vi "Low Over Current Test 1.vi"(0 "Device Name":string="Dev4", 1 "Device/Ports/Lines":string="Dev1/port0/line1,Dev1/port0/line13,Dev1/port0/line6,Dev1/port0/line23,Dev1/port0/line17", 3 "error in":errorcluster) -> (10 "error out":errorcluster)   [LabVIEW 2015]
panel:
  # "True means close relay"
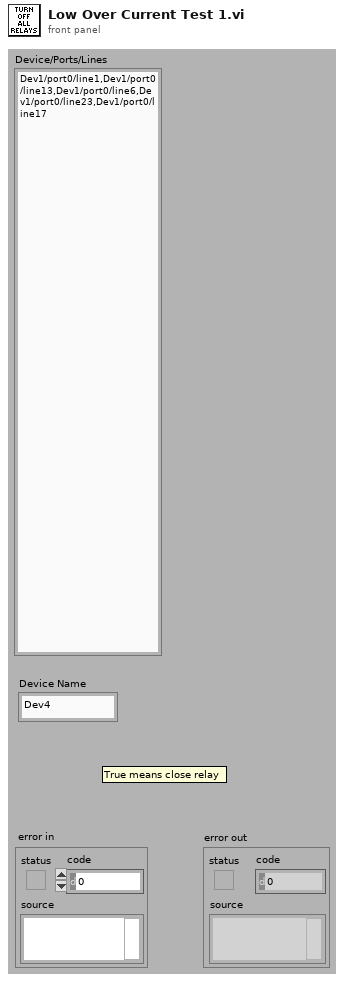
[diagram p1: front panel]
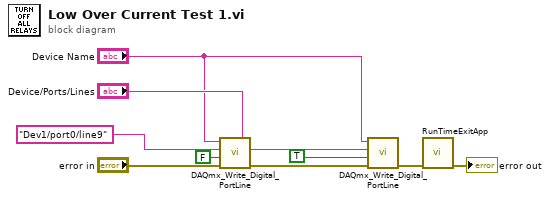
[diagram p0: block diagram]
diagram:
  n1 = call "DAQmx_Write_Digital_PortLine.vi"("Device/Ports/Lines"="Device Name", 1:"Dev1/port0/line9" ("Device/Ports/Lines"), "Boolean"=FALSE, "error in"="error in") -> ("error out"=w5:errorcluster)  [unwired: 5 in, 1 out]
  n2 = call "DAQmx_Write_Digital_PortLine.vi"("Device/Ports/Lines"="Device Name", 1:"Device/Ports/Lines", "Boolean"=TRUE, "error in"=w5) -> ("error out"=w7:errorcluster)  [unwired: 5 in, 1 out]
  n3 = call "RunTimeExitApp.vi"("error in (no error)"=w7) -> ("error out"=→"error out":errorcluster)  [unwired: 10 in]
